vi "SRV_Motor Button - Get Button Name.vi"(5 "Number of Columns":i32=7, 9 "Index":i32) -> (8 "Button Name":string)   [LabVIEW 2014]
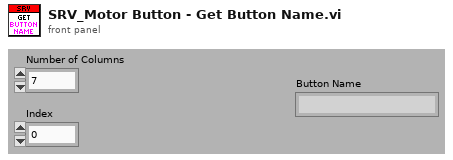
[diagram p1: front panel]
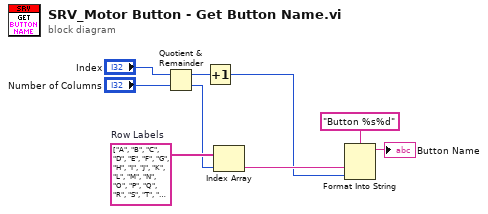
[diagram p0: block diagram]
diagram:
  w9 = string[] ["A", "B", "C", "D", "E", "F", "G", "H", "I", "J", "K", "L", "M", "N", "O", "P", "Q", "R", "S", "T", "U", "V", "W", "X", "Y", "Z"]  # Row Labels
  n1 = Quotient & Remainder(x="Index", y="Number of Columns") -> (x-y*floor(x/y)=w7:i32, floor(x/y)=w6:i32)
  n2 = Increment(x=w7) -> (x+1=w4:i32)
  n3 = Index Array(array=w9, index=w6) -> (element=w5:string)
  n4 = Format Into String(format string="Button %s%d", w5, w4) -> (resulting string=→"Button Name":string)  [unwired: 2 in, 1 out]
